vi "CTI_AOTF-configure.vi"(9 "error out":errorcluster, 10 "CTI-AOTF":T1, 11 "check-online":bool[](array[boolean])) -> ()   [LabVIEW 2011]
panel:
  in  "Power / [%] 8":i16 min=0 max=100 step=1
  in  "Power / [%] 7":i16 min=0 max=100 step=1
  in  "Power / [%] 6":i16 min=0 max=100 step=1
  in  "Power / [%] 5":i16 min=0 max=100 step=1
  in  "Power / [%] 4":i16 min=0 max=100 step=1
  in  "Power / [%] 3":i16 min=0 max=100 step=1
  in  "Power / [%] 2":i16 min=0 max=100 step=1
  in  "Power / [%]":i16 min=0 max=100 step=1
  in  "Boolean":bool
  in  "Boolean 2":bool
  in  "Boolean 3":bool
  in  "Boolean 4":bool
  in  "Boolean 5":bool
  in  "Boolean 6":bool
  in  "Boolean 7":bool
  in  "Boolean 8":bool
  in  "Numeric 8":i32=490 min=490 max=730 step=1
  in  "Numeric":i32=490 min=490 max=730 step=1
  in  "Numeric 2":i32=490 min=490 max=730 step=1
  in  "Numeric 3":i32=490 min=490 max=730 step=1
  in  "Numeric 4":i32=490 min=490 max=730 step=1
  in  "Numeric 5":i32=490 min=490 max=730 step=1
  in  "Numeric 6":i32=490 min=490 max=730 step=1
  in  "Numeric 7":i32=490 min=490 max=730 step=1
  in  "Combo Box 2":string(combo)="490"
  in  "Combo Box 3":string(combo)="490"
  in  "Combo Box 4":string(combo)="490"
  in  "Combo Box 5":string(combo)="490"
  in  "Combo Box 6":string(combo)="490"
  in  "Combo Box 7":string(combo)="490"
  in  "Combo Box 8":string(combo)="490"
  in  "Combo Box 9":string(combo)="490"
  in  "Radio Buttons":enum32{"Radio Selection 1", "Radio Selection 2"}(radio)
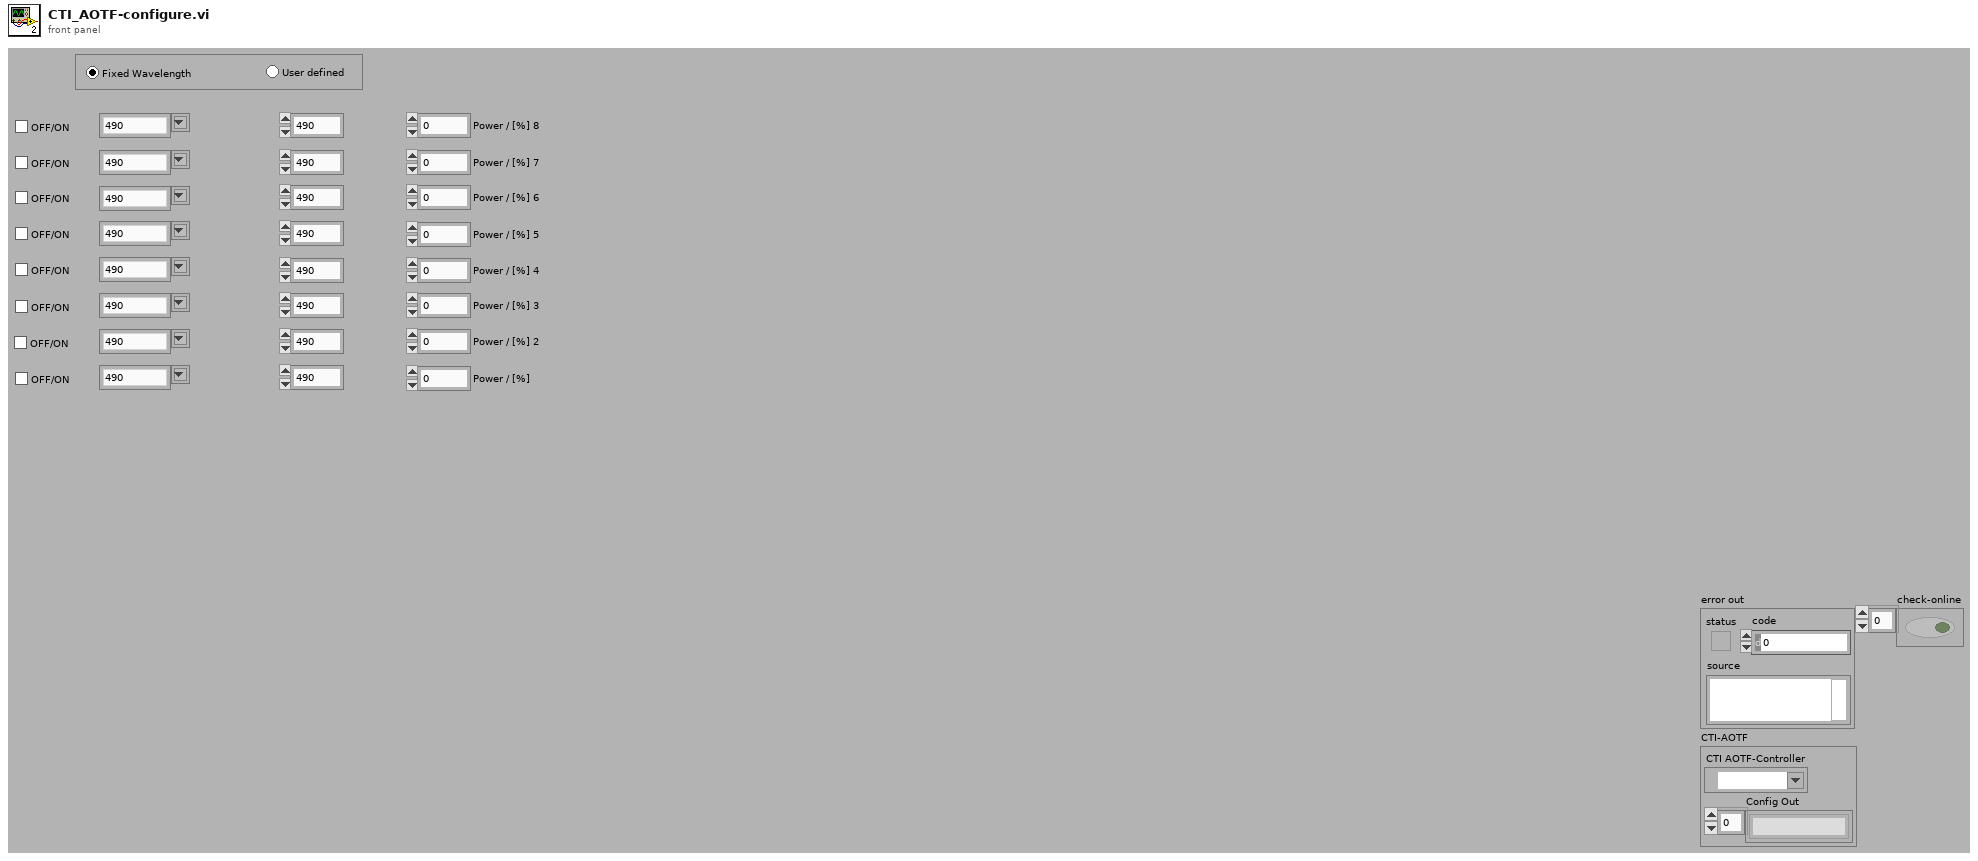
[diagram p1: front panel]
types:
  T1 = cluster{"CTI AOTF-Controller":refnum<visa-resource-name>, "Config Out":string[]}
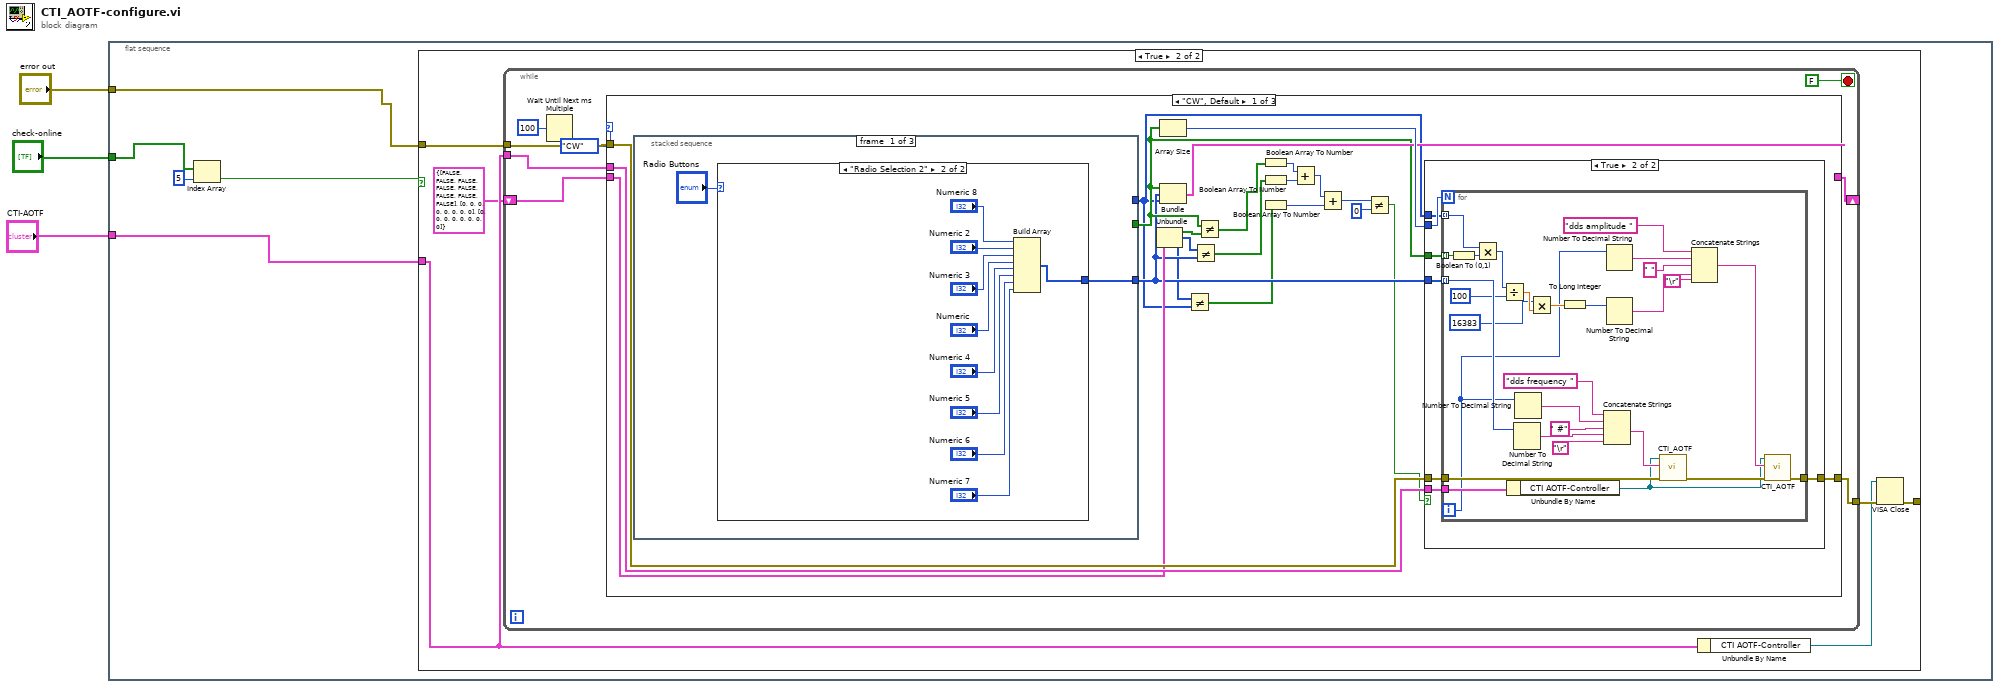
[diagram p0: block diagram]
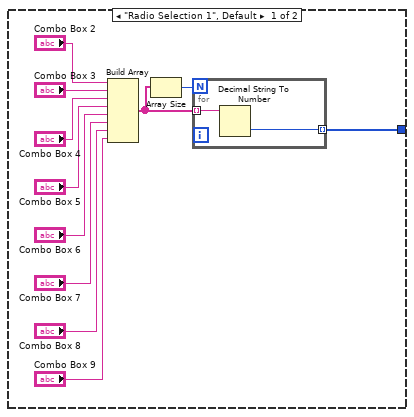
[diagram p4: hidden frame]
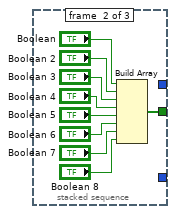
[diagram p5: hidden frame]
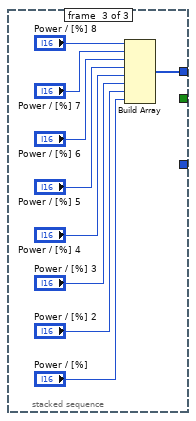
[diagram p6: hidden frame]
diagram:
  n1 = flat-sequence {
    tunnel: "error out" -> [w6]
    tunnel: "check-online" -> [w5]
    tunnel: "CTI-AOTF" -> [w4]
    frame #0 {
      n2 = Index Array(array=w5, index=5) -> (element=w7:bool)
      n3 = case shown="True" w7 {
        tunnel: w6 -> [w9 w15]
        tunnel: w4 -> [_ w11]
        tunnel: [w9 w12] -> _
        frame False {
        }
        frame True {
          n4 = while {
            shift-right: [w22] -> _
            shift-left: cluster{bool[], i32[], i16[]} {[FALSE, FALSE, FALSE, FALSE, FALSE, FALSE, FALSE, FALSE], [0, 0, 0, 0, 0, 0, 0, 0], [0, 0, 0, 0, 0, 0, 0, 0]} -> [w21]
            tunnel: w15 -> [w20]
            tunnel: [w19] -> w14
            tunnel: w11 -> [w18]
            stop <- FALSE stop-if-true
            n5 = Wait Until Next ms Multiple(millisecond multiple=u32 100) -> ()  [unwired: 1 out]
            n6 = case shown="\"CW\", Default" enum32{"CW", "Pulsed", "Ramp"}."CW" ("Value") {
              tunnel: [w44 w125 w126] -> w22
              tunnel: w21 -> [w34 w125 w126]
              tunnel: w20 -> [w37 w124 w127]
              tunnel: [w36 w124 w127] -> w19
              tunnel: w18 -> [w35 _ _]
              frame "CW", Default {
                n7 = stacked-sequence {
                  tunnel: [w83 _ _] -> w31
                  tunnel: [_ w106 _] -> w33
                  tunnel: [_ _ w115] -> w29
                  frame #0 {
                    n8 = case shown="\"Radio Selection 2\"" "Radio Buttons" {
                      tunnel: [w84 w97] -> w83
                      frame "Radio Selection 1", Default {
                        n9 = Build Array("Combo Box 2", "Combo Box 3", "Combo Box 4", "Combo Box 5", "Combo Box 6", "Combo Box 7", "Combo Box 8", "Combo Box 9") -> (w86:string[])
                        n10 = Array Size(array=w86) -> (size(s)=w85:i32)
                        n11 = for {
                          N: w85 -> [_]
                          tunnel: w86 -> [w96] mode=indexing
                          tunnel: [w95] -> w84 mode=indexing
                          n12 = Decimal String To Number(string=w96) -> (number=w95:i32)  [unwired: 2 in, 1 out]
                        }
                      }
                      frame "Radio Selection 2" {
                        n13 = Build Array("Numeric 8", "Numeric 2", "Numeric 3", "Numeric", "Numeric 4", "Numeric 5", "Numeric 6", "Numeric 7") -> (w97:i32[])
                      }
                    }
                  }
                  frame #1 {
                    n14 = Build Array("Boolean", "Boolean 2", "Boolean 3", "Boolean 4", "Boolean 5", "Boolean 6", "Boolean 7", "Boolean 8") -> (w106:bool[])
                  }
                  frame #2 {
                    n15 = Build Array("Power / [%] 8", "Power / [%] 7", "Power / [%] 6", "Power / [%] 5", "Power / [%] 4", "Power / [%] 3", "Power / [%] 2", "Power / [%]") -> (w115:i16[])
                  }
                }
                n16 = Unbundle(w34) -> (w32:bool[], w30:i32[], w28:i16[])
                n17 = Array Size(array=w33) -> (size(s)=w45:i32)
                n18 = Bundle(w33, w31, w29) -> (w44:cluster{bool[], i32[], i16[]})  [unwired: 1 in]
                n19 = Not Equal?(x=w28, y=w29) -> (x != y?=w25:bool[])
                n20 = Not Equal?(x=w30, y=w31) -> (x != y?=w26:bool[])
                n21 = Not Equal?(x=w33, y=w32) -> (x != y?=w27:bool[])
                n22 = Boolean Array To Number(Boolean array=w27) -> (number=w43:u32)
                n23 = Boolean Array To Number(Boolean array=w26) -> (number=w42:u32)
                n24 = Boolean Array To Number(Boolean array=w25) -> (number=w40:u32)
                n25 = Add(x=w43, y=w42) -> (x+y=w41:u32)
                n26 = Add(x=w41, y=w40) -> (x+y=w39:u32)
                n27 = Not Equal?(x=w39, y=u32 0) -> (x != y?=w24:bool)
                n28 = case shown="True" w24 {
                  tunnel: w45 -> [_ w53]
                  tunnel: w33 -> [_ w52]
                  tunnel: w31 -> [_ w51]
                  tunnel: w29 -> [_ w50]
                  tunnel: w37 -> [w46 w49]
                  tunnel: [w46 w48] -> w36
                  tunnel: w35 -> [_ w47]
                  frame False {
                  }
                  frame True {
                    n29 = for {
                      N: w53 -> [_]
                      tunnel: w52 -> [w63] mode=indexing
                      tunnel: w51 -> [w73] mode=indexing
                      tunnel: w50 -> [w61] mode=indexing
                      tunnel: w49 -> [w81]
                      tunnel: [w57] -> w48
                      tunnel: w47 -> [w80]
                      i -> [w54]
                      n30 = Boolean To (0,1)(Boolean=w63) -> (0, 1=w62:i16)
                      n31 = Multiply(x=w61, y=w62) -> (x*y=w60:i16)
                      n32 = Divide(x=w60, y=100) -> (x/y=w70:dbl)
                      n33 = Unbundle By Name(w80) -> ("CTI AOTF-Controller"=w55:refnum<visa-resource-name>)
                      n34 = Number To Decimal String(number=w73) -> (decimal integer string=w76:string)  [unwired: 1 out]
                      n35 = Number To Decimal String(number=w54) -> (decimal integer string=w78:string)  [unwired: 1 out]
                      n36 = Multiply(x=16383, y=w70) -> (x*y=w68:dbl)
                      n37 = To Long Integer(number=w68) -> (32bit integer=w64:i32)
                      n38 = Concatenate Strings("dds frequency " ("string"), w78, " #" ("string"), w76, "\r") -> (w74:string)
                      n39 = Number To Decimal String(number=w54) -> (decimal integer string=w72:string)  [unwired: 1 out]
                      n40 = Number To Decimal String(number=w64) -> (decimal integer string=w66:string)  [unwired: 1 out]
                      n41 = call "CTI_AOTF.vi"("error in"=w81, "String"=w74, "VISA resource name 2"=w55) -> ("error out"=w58:errorcluster)  [unwired: 7 in, 1 out]
                      n42 = Concatenate Strings("dds amplitude " ("string"), w72, " " ("string"), w66, "\r") -> (w56:string)
                      n43 = call "CTI_AOTF.vi"("error in"=w58, "String"=w56, "VISA resource name 2"=w55) -> ("error out"=w57:errorcluster)  [unwired: 7 in, 1 out]
                    }
                  }
                }
              }
              frame "Pulsed" {
              }
              frame "Ramp" {
              }
            }
          }
          n44 = Unbundle By Name(w11) -> ("CTI AOTF-Controller"=w13:refnum<visa-resource-name>)
          n45 = VISA Close(VISA resource name=w13, error in (no error)=w14) -> (error out=w12:errorcluster)
        }
      }
    }
  }
